vi "New dotNET WebSocket Server.vi"(7 "Server SSL Options (wss://)":T1={"Check Revocation"=FALSE, "Client Cert Required"=FALSE, "Server Certificate"={"PFX Certificate"=path "", "PFX Password"=""}, "SSL Protocols"=[240]} {"SSL Protocols" items=["None"=0, "Ssl2"=12, "Ssl3"=48, "Tls"=192, "Default"=240, "Tls11"=768, "Tls12"=3072]}, 8 "error in (no error)":errorcluster, 9 "Timeout (5000ms)":i32=5000, 10 "Use SSL?":bool, 11 "Socket in":refnum<class "Socket.lvclass">) -> (0 "error out":errorcluster, 3 "dotNET WebSocket Server out":refnum<class "dotNET WebSocket Server.lvclass">)   [LabVIEW 2013, in "dotNET WebSocket.lvlib" / "dotNET WebSocket Server.lvclass"]
doc: "Creates a new WebSocket Server connection using dotNET from the dotNET listener functions. Supports ws:// and wss:// protocols."
uses:
  dotNET WebSocket Server.lvclass
  <vilib>/MediaMongrels Ltd/WebSockets/Sockets/Socket/Socket.lvclass
  Server SSL Options.ctl
  dotNET SSL Socket/PFX Certificate.ctl
  dotNET SSL Socket/dotNET SSL Socket.lvclass/dotNET SSL Socket.ctl
  dotNET SSL Server/dotNET SSL Server.lvclass/dotNET SSL Server.ctl
  dotNET SSL Server/dotNET SSL Server.lvclass
  <vilib>/MediaMongrels Ltd/WebSockets/WebSockets/WebSocket/WebSocket.lvclass/WebSocket.ctl
  dotNET SSL Socket/Write Check Revocation.vi
  dotNET SSL Server/Write Client Cert Required.vi
  dotNET SSL Socket/Write SSL Protocols.vi
  dotNET SSL Server/Write Server Certificate.vi
  <vilib>/MediaMongrels Ltd/WebSockets/WebSockets/WebSocket/Write Socket.vi
  dotNET SSL Socket/dotNET SSL Socket.lvclass
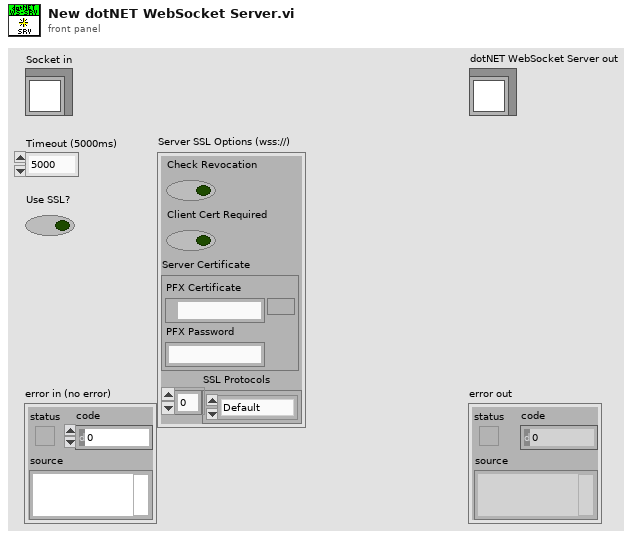
[diagram p1: front panel]
types:
  T1 = typedef "dotNET WebSocket.lvlib/dotNET WebSocket Server.lvclass/Server SSL Options.ctl" = cluster{"Check Revocation":bool, "Client Cert Required":bool, "Server Certificate":T2, "SSL Protocols":i32[]}
  T2 = typedef "dotNET SSL Socket.lvlib/dotNET SSL Socket.lvclass/PFX Certificate.ctl" = cluster{"PFX Certificate":path, "PFX Password":string}
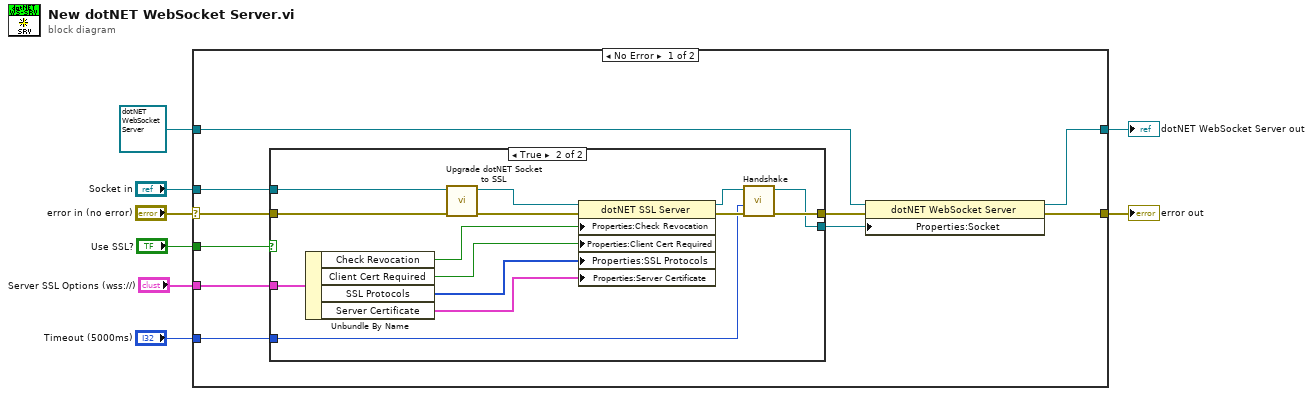
[diagram p0: block diagram]
diagram:
  n1 = case shown="No Error" "error in (no error)" {
    selector: "error in (no error)" -> [w13 w36]
    tunnel: [w12 w36] -> w7
    tunnel: [w11 w35] -> w6
    tunnel: refnum<class "dotNET WebSocket Server.lvclass"> refnum ("dotNET WebSocket.lvlib:dotNET WebSocket Server") -> [w18 w35]
    tunnel: "Timeout (5000ms)" -> [w15 _]
    tunnel: "Socket in" -> [w14 _]
    tunnel: "Use SSL?" -> [w10 _]
    tunnel: "Server SSL Options (wss://)" -> [w9 _]
    frame No Error {
      n2 = case shown="True" w10 {
        tunnel: [w19 w30] -> w17
        tunnel: [w20 w29] -> w16
        tunnel: w15 -> [_ w28]
        tunnel: w14 -> [w20 w27]
        tunnel: w13 -> [w19 w26]
        tunnel: w9 -> [_ w25]
        frame False {
        }
        frame True {
          n3 = Unbundle By Name(w25) -> ("Check Revocation"=w24:bool, "Client Cert Required"=w23:bool, "SSL Protocols"=w22:i32[], "Server Certificate"=w21:T2)
          n4 = call "Upgrade dotNET Socket to SSL.vi"("error in (no error)"=w26, "Socket in"=w27) -> ("error out"=w34:errorcluster, "dotNET SSL Socket out"=w32:refnum<class "dotNET SSL Server.lvclass">)  [unwired: 8 in]
          n5 = property class="dotNET SSL Server"(reference=w32, error in=w34, "Properties:Check Revocation"=w24, "Properties:Client Cert Required"=w23, "Properties:SSL Protocols"=w22, "Properties:Server Certificate"=w21) -> (reference out=w31:refnum<class "dotNET SSL Server.lvclass">, error out=w33:errorcluster)
          n6 = call-dynamic "Handshake.vi"("error in (no error)"=w33, "Timeout (5000ms)"=w28, "dotNET SSL Socket in"=w31) -> ("error out"=w30:errorcluster, "dotNET SSL Socket out"=w29:refnum<class "dotNET SSL Server.lvclass">)  [unwired: 7 in]
        }
      }
      n7 = property class="dotNET WebSocket Server"(reference=w18, error in=w17, "Properties:Socket"=w16) -> (reference out=w11:refnum<class "dotNET WebSocket Server.lvclass">, error out=w12:errorcluster)
    }
    frame Error {
    }
  }
  "error out" <- w7
  "dotNET WebSocket Server out" <- w6
